vi "Unflatten Variant from JSON.vi"(8 "error in (no error)":errorcluster, 11 "JSON String":string) -> (0 "error out":errorcluster, 3 "JSON Value out":variant)   [LabVIEW 2017, in "Advanced Variant Tools.lvlib" / "JSON Support.lvlib"]
doc: "Unflattens the given JSON string to a JSON instance"
uses:
  JSON Support.lvlib
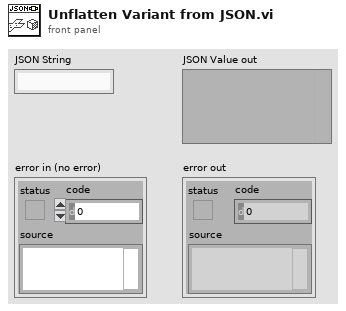
[diagram p1: front panel]
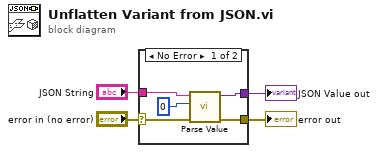
[diagram p0: block diagram]
diagram:
  n1 = case shown="No Error" "error in (no error)" {
    selector: "error in (no error)" -> [w9 w10]
    tunnel: [w7 w10] -> w2
    tunnel: [w8 _] -> w3
    tunnel: "JSON String" -> [w6 _]
    frame No Error {
      n2 = call "Parse Value.vi"("error in (no error)"=w9, "Index In"=0, "JSON String"=w6) -> ("error out"=w7:errorcluster, "JSON Value out"=w8:variant)  [unwired: 6 in, 1 out]
    }
    frame Error {
    }
  }
  "error out" <- w2
  "JSON Value out" <- w3
